vi "ArrayToExcel.vi"() -> ()   [LabVIEW 2020]
uses:
  <vilib>/Analysis/NI_AALBase.lvlib
panel:
  out "Tabla":string[][](array[string])
  out "Waveform Graph":dbl[][](graph)
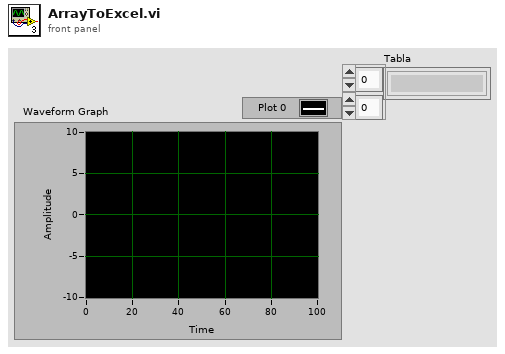
[diagram p1: front panel]
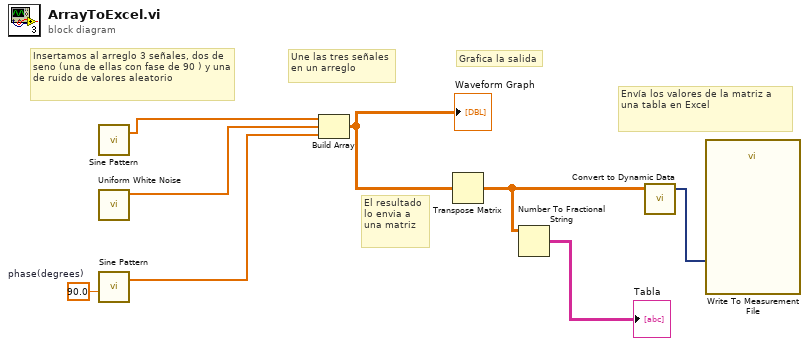
[diagram p0: block diagram]
diagram:
  w8 = 90.0  # phase(degrees)
  # "Envía los valores de la matriz a una tabla en Excel"
  # "El resultado lo envia a una matriz"
  # "Grafica la salida"
  # "Une las tres señales en un arreglo"
  # "Insertamos al arreglo 3 señales, dos de seno (una de ellas con fase de 90 ) y una de ruido de valores aleatorio"
  n1 = call <vilib>:"Sine Pattern.vi"() -> ("Sinusoidal Pattern"=w7:dbl[])  [unwired: 4 in, 1 out]
  n2 = call <vilib>:"Uniform White Noise.vi"() -> ("uniform white noise"=w6:dbl[])  [unwired: 10 in, 1 out]
  n3 = call <vilib>:"Sine Pattern.vi"("phase(degrees)"=w8) -> ("Sinusoidal Pattern"=w5:dbl[])  [unwired: 3 in, 1 out]
  n4 = Build Array "Build Array"(w7, w6, w5) -> (w4:dbl[][])
  "Waveform Graph" <- w4
  n5 = Transpose Matrix(1:w4) -> (0:w2:dbl[][])
  n6 = Number To Fractional String(number=w2) -> (F-format string=→"Tabla":string[][])  [unwired: 3 in]
  n7 = call "Convert to Dynamic Data"("2D Array"=w2) -> ("Dynamic Data Type"=w1:dynamicdata)  [unwired: 3 in]
  n8 = call "Write To Measurement File"("Signals"=w1) -> ()  [unwired: 16 in, 3 out]
